vi "MAKE DISPLAY ARRAY.vi"(3 "VNA DATA CLUSTER":T1, 4 "PERSISTANCE DATA CLUSTER":T1, 5 "Display type (F : MAG/PHASE)":bool, 6 "Persistance":bool) -> (1 "Display array":T2(array[cluster]))   [LabVIEW 2021]
uses:
  Spectrum data.ctl
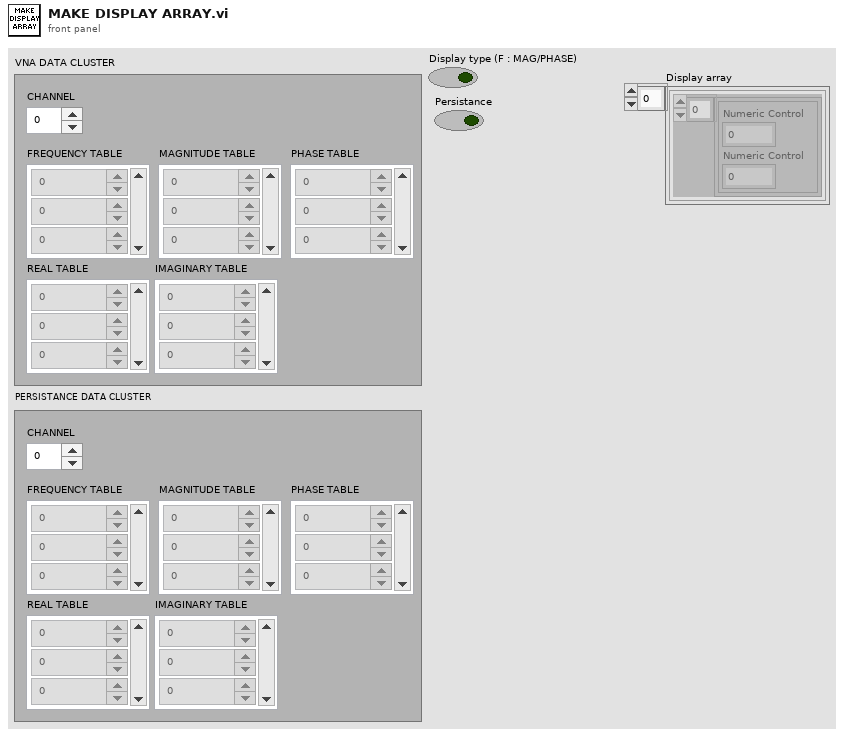
[diagram p1: front panel]
types:
  T1 = typedef "Spectrum data.ctl" = cluster{"CHANNEL":dbl, "FREQUENCY TABLE":ext[], "MAGNITUDE TABLE":ext[], "PHASE TABLE":ext[], "REAL TABLE":ext[], "IMAGINARY TABLE":ext[]}
  T2 = cluster{cluster{"Numeric Control":ext, "Numeric Control":ext}[]}[]
  T3 = cluster{"Numeric Control":ext, "Numeric Control":ext}[]
  T4 = cluster{cluster{"Numeric Control":ext, "Numeric Control":ext}[]}
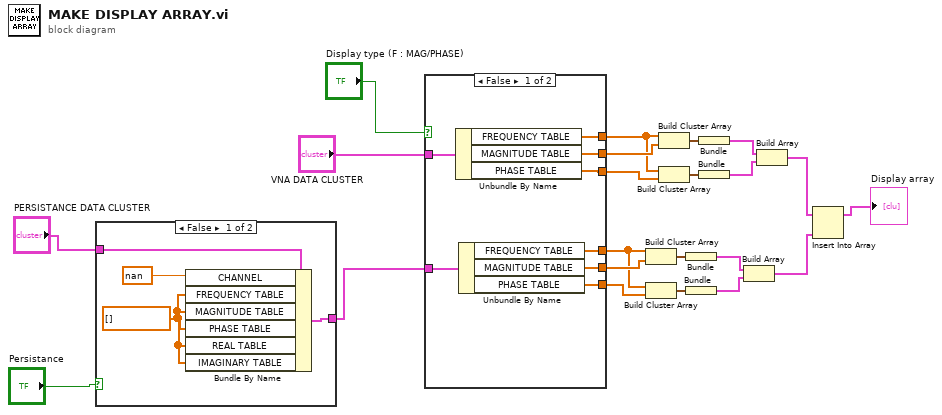
[diagram p0: block diagram]
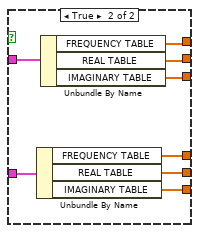
[diagram p3: hidden frame]
diagram:
  n1 = case shown="False" "Persistance" {
    tunnel: "PERSISTANCE DATA CLUSTER" -> [w26 w27]
    tunnel: [w25 w27] -> w11
    frame False {
      w23 = dbl[] [] ("FREQUENCY TABLE")
      n2 = Bundle By Name(cluster=w26, "CHANNEL"=nan, "FREQUENCY TABLE"=w23, "MAGNITUDE TABLE"=w23, "PHASE TABLE"=w23, "REAL TABLE"=w23, "IMAGINARY TABLE"=w23) -> (w25:T1)
    }
    frame True {
    }
  }
  n3 = case shown="False" "Display type (F : MAG/PHASE)" {
    tunnel: [w35 w41] -> w18
    tunnel: [w34 w42] -> w17
    tunnel: [w33 w40] -> w16
    tunnel: "VNA DATA CLUSTER" -> [w32 w43]
    tunnel: w11 -> [w31 w39]
    tunnel: [w30 w38] -> w5
    tunnel: [w29 w37] -> w6
    tunnel: [w28 w36] -> w4
    frame False {
      n4 = Unbundle By Name(w32) -> ("FREQUENCY TABLE"=w34:ext[], "MAGNITUDE TABLE"=w35:ext[], "PHASE TABLE"=w33:ext[])
      n5 = Unbundle By Name(w31) -> ("FREQUENCY TABLE"=w30:ext[], "MAGNITUDE TABLE"=w29:ext[], "PHASE TABLE"=w28:ext[])
    }
    frame True {
      n6 = Unbundle By Name(w39) -> ("FREQUENCY TABLE"=w38:ext[], "REAL TABLE"=w37:ext[], "IMAGINARY TABLE"=w36:ext[])
      n7 = Unbundle By Name(w43) -> ("FREQUENCY TABLE"=w42:ext[], "REAL TABLE"=w41:ext[], "IMAGINARY TABLE"=w40:ext[])
    }
  }
  n8 = Build Cluster Array(w5, w6) -> (w9:T3)
  n9 = Build Cluster Array(w5, w4) -> (w10:T3)
  n10 = Build Cluster Array(w17, w18) -> (w21:T3)
  n11 = Build Cluster Array(w17, w16) -> (w22:T3)
  n12 = Bundle(w9) -> (w8:T4)  [unwired: 1 in]
  n13 = Bundle(w10) -> (w7:T4)  [unwired: 1 in]
  n14 = Bundle(w21) -> (w20:T4)  [unwired: 1 in]
  n15 = Bundle(w22) -> (w19:T4)  [unwired: 1 in]
  n16 = Build Array(w8, w7) -> (w2:T2)
  n17 = Build Array(w20, w19) -> (w3:T2)
  n18 = Insert Into Array(array=w3, new element=w2) -> (→"Display array":T2)  [unwired: 1 in]
